vi "Read Index Values.vi"(8 "error in (no error)":errorcluster, 11 "Array.lvclass in":refnum<class "Array.lvclass">) -> (0 "error out":errorcluster, 2 "IndexVals":u32[](array[numeric]), 3 "Array.lvclass out":refnum<class "Array.lvclass">)   [LabVIEW 2015, in "Array.lvclass"]
uses:
  Array.lvclass
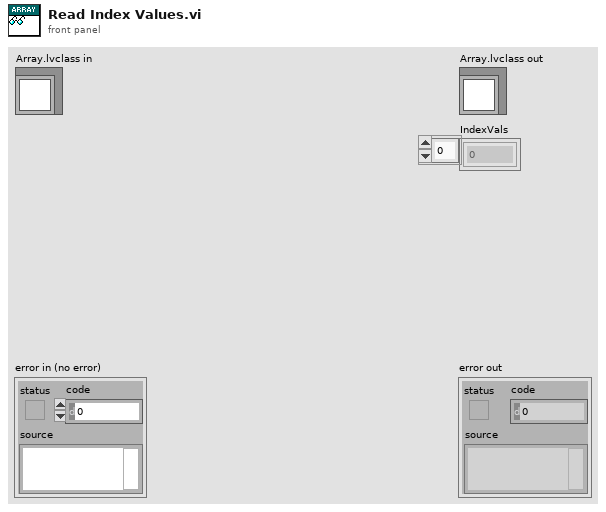
[diagram p1: front panel]
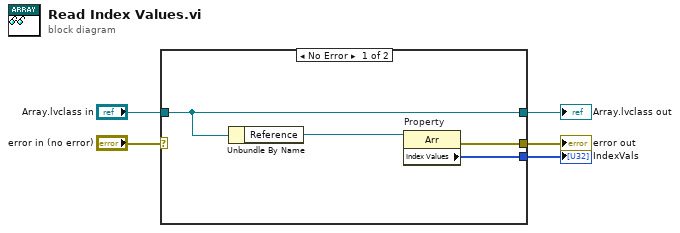
[diagram p0: block diagram]
diagram:
  n1 = case shown="No Error" "error in (no error)" {
    selector: "error in (no error)" -> [_ w11]
    tunnel: [w8 w11] -> w4
    tunnel: [w7 w10] -> w2
    tunnel: "Array.lvclass in" -> [w7 w10]
    tunnel: [w9 _] -> w1
    frame No Error {
      n2 = Unbundle By Name(w7) -> ("Reference"=w6:refnum<vi>)
      n3 = property on="Property" class="Arr"(reference=w6) -> (error out=w8:errorcluster, "Index Values"=w9:u32[])  [unwired: 1 in, 1 out]
    }
    frame Error {
    }
  }
  "error out" <- w4
  "Array.lvclass out" <- w2
  "IndexVals" <- w1
